vi "Lester Roche Programacion 4 (2).vi"() -> ()   [LabVIEW 2011]
panel:
  out "Rango":string
  out "121-180":bool
  out "81-120":bool
  out "1-80":bool
  out "Velocidad":dbl(knob) scale=0.0..180.0
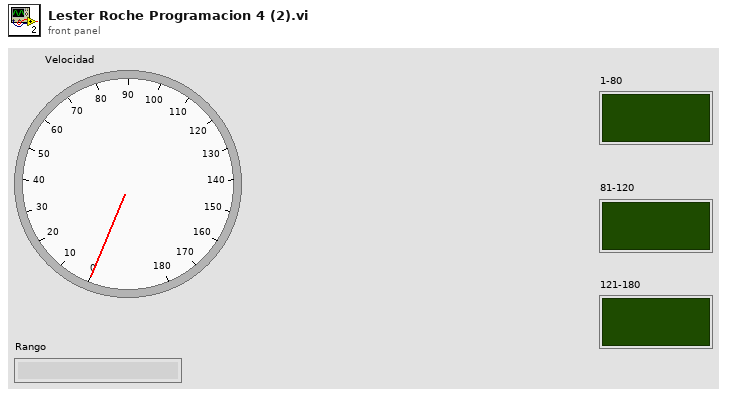
[diagram p1: front panel]
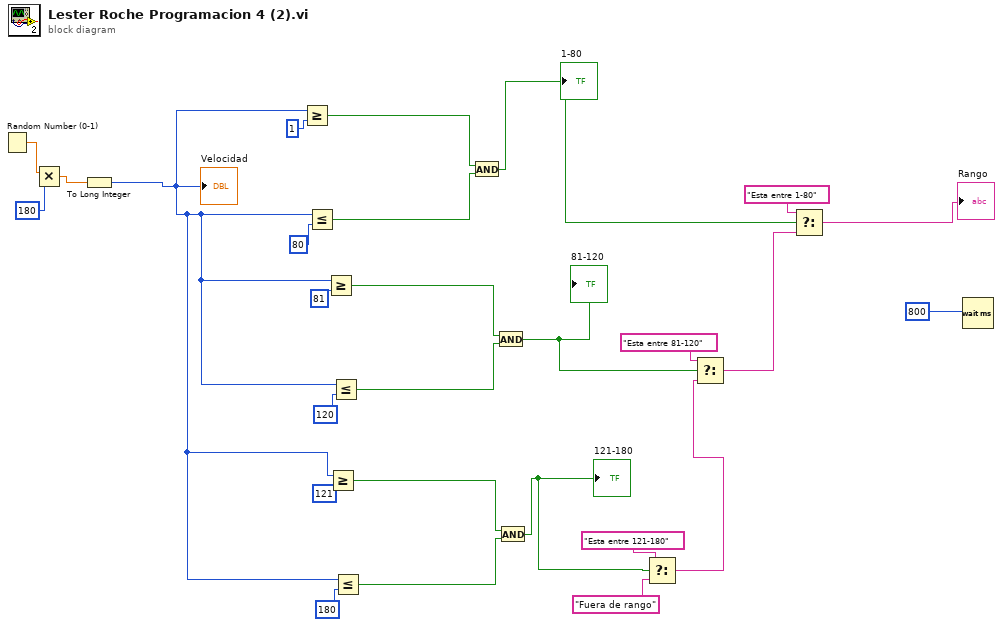
[diagram p0: block diagram]
diagram:
  n1 = Random Number (0-1)() -> (number: 0 to 1=w26:dbl)
  n2 = Multiply(x=w26, y=180) -> (x*y=w25:dbl)
  n3 = To Long Integer(number=w25) -> (32bit integer=w12:i32)
  "Velocidad" <- w12
  n4 = Greater Or Equal?(x=w12, y=1) -> (x >= y?=w22:bool)
  n5 = Less Or Equal?(x=w12, y=80) -> (x <= y?=w21:bool)
  n6 = Greater Or Equal?(x=w12, y=81) -> (x >= y?=w19:bool)
  n7 = Greater Or Equal?(x=w12, y=121) -> (x >= y?=w14:bool)
  n8 = Less Or Equal?(x=w12, y=120) -> (x <= y?=w20:bool)
  n9 = Less Or Equal?(x=w12, y=180) -> (x <= y?=w13:bool)
  n10 = And(x=w22, y=w21) -> (x .and. y?=w10:bool)
  "1-80" <- w10
  n11 = And(x=w19, y=w20) -> (x .and. y?=w7:bool)
  "81-120" <- w7
  n12 = And(x=w14, y=w13) -> (x .and. y?=w4:bool)
  "121-180" <- w4
  n13 = Select(t="Esta entre 121-180", s=w4, f="Fuera de rango") -> (s? t:f=w3:string)
  n14 = Select(t="Esta entre 81-120", s=w7, f=w3) -> (s? t:f=w6:string)
  n15 = Select(t="Esta entre 1-80", s=w10, f=w6) -> (s? t:f=→"Rango":string)
  n16 = Wait (ms)(milliseconds to wait=800) -> ()  [unwired: 1 out]
